vi "Auto State Machine.vi"   [LabVIEW 2013]
uses:
  typedefs/fg_typedef.ctl
  typedefs/State Machine/singleUseSubstate.ctl
  typedefs/Vision/vision enable.ctl
  typedefs/DevRef Type.ctl
  typedefs/State Machine/subStates.ctl
panel:
  # "A State Machine to Handle One or Two Ball Autonomous"
types:
  T1 = typedef "fg_typedef.ctl" = enum16{"Get", "Set"}
  T2 = typedef "subStates.ctl" = enum16{"null", "wait", "driver control", "auto", "manual override", "hold position", "rotate", "pickup", "pass", "recover pass", "load", "goto shoot", "shoot high goal", "shoot low goal", "cancel arm", "cancel shooter", "end", "test"}
  T3 = typedef "singleUseSubstate.ctl" = enum16{"null", "wait", "shift high", "shift low", "extend shooter", "retract shooter", "latch", "unlatch", "end"}
  T4 = typedef "vision enable.ctl" = enum16{"Enable", "Disable", "Stop"}
  T5 = typedef "DevRef Type.ctl" = enum16{"Shooter Solenoid", "Latch Solenoid", "Right Up Sensor", "Right Down Sensor", "Hold Sensor", "Arm Encoder"}
  T6 = typedef "WPI_EncoderDevRef.ctl" = cluster{"DevStatus":errorcluster, "EncoderIndex":T7, "CounterIndex":T8, "DistancePerCount":dbl, "Decoding Type":T9}
  T7 = typedef "FPGA_EncoderIdx.ctl" = enum8{"Enc 0", "Enc 1", "Enc 2", "Enc 3", "Invalid"}
  T8 = typedef "FPGA_CounterCtrSystemIndex.ctl" = enum8{"Ctr 0", "Ctr 1", "Ctr 2", "Ctr 3", "Ctr 4", "Ctr 5", "Ctr 6", "Ctr 7", "Invalid"}
  T9 = typedef "WPI_EncoderType.ctl" = enum16{"1x", "2x", "4x"}
  T10 = typedef "WPI_DigitalInputDevRef.ctl" = cluster{"DevStatus":errorcluster, "DIO Channel":T11, "Digital Module":T12}
  T11 = typedef "FPGA_DIOChannel.ctl" = enum8{"DIO 1", "DIO 2", "DIO 3", "DIO 4", "DIO 5", "DIO 6", "DIO 7", "DIO 8", "DIO 9", "DIO 10", "DIO 11", "DIO 12", "DIO 13", "DIO 14", "Invalid"}
  T12 = typedef "FPGA_TypedefDigitalModule.ctl" = enum16{"Digital Module 1", "Digital Module 2"}
  T13 = typedef "vision data.ctl" = cluster{"x":dbl, "y":dbl, "area":dbl, "width":dbl, "height":dbl, "Hot Goal Present?":bool, "distance":dbl}
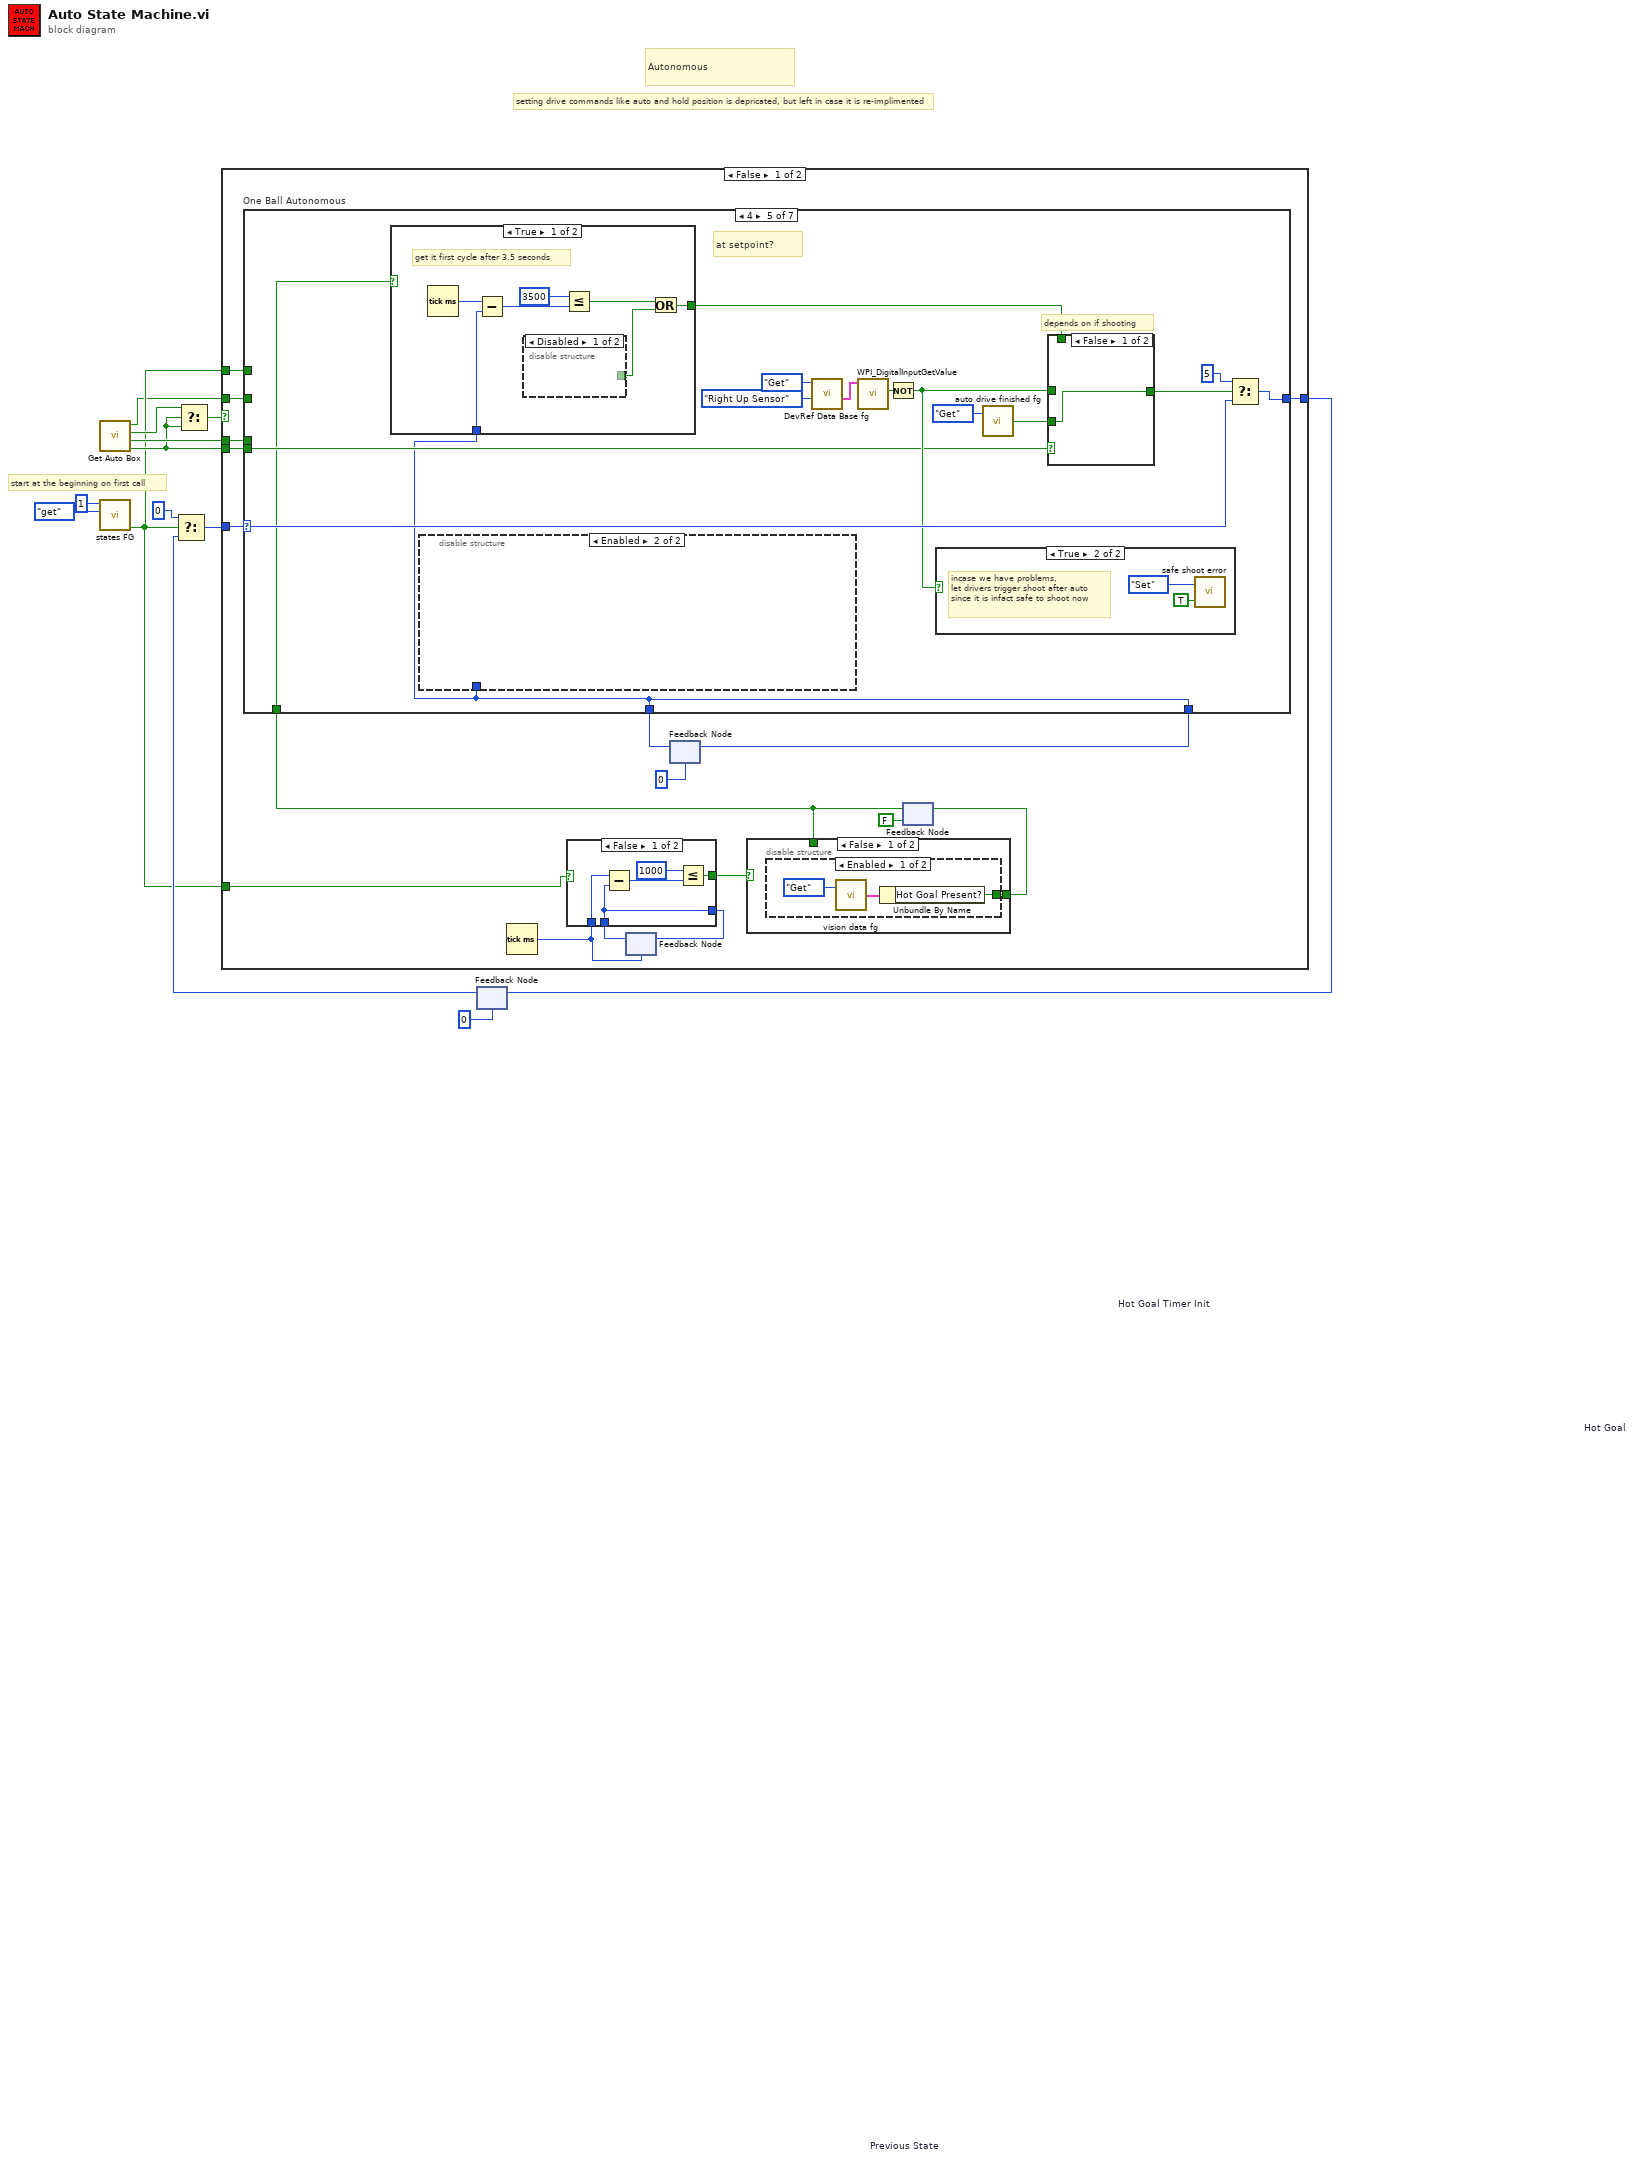
[diagram p0: block diagram]
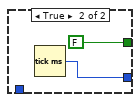
[diagram p2: hidden frame]
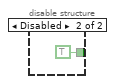
[diagram p3: hidden frame]
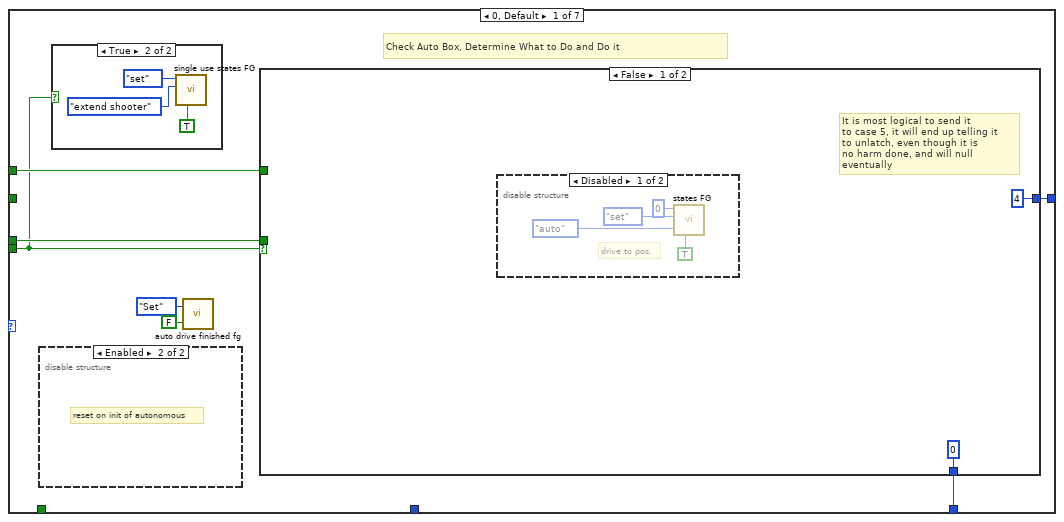
[diagram p5: hidden frame]
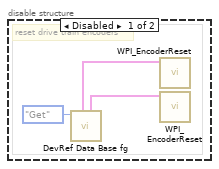
[diagram p6: hidden frame]
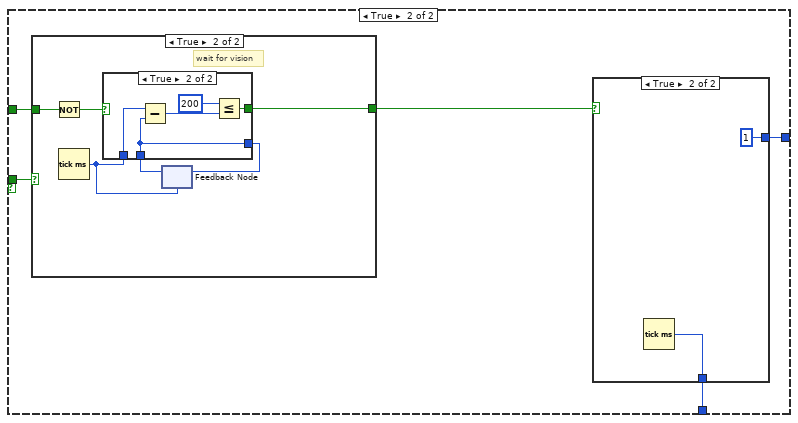
[diagram p8: hidden frame]
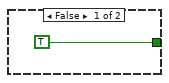
[diagram p9: hidden frame]
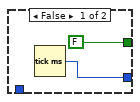
[diagram p10: hidden frame]
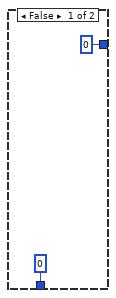
[diagram p11: hidden frame]
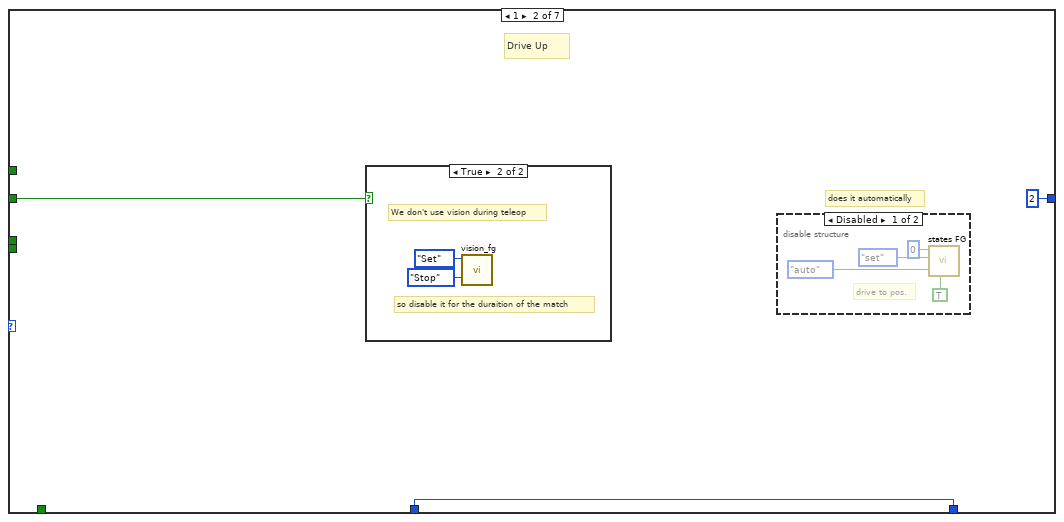
[diagram p13: hidden frame]
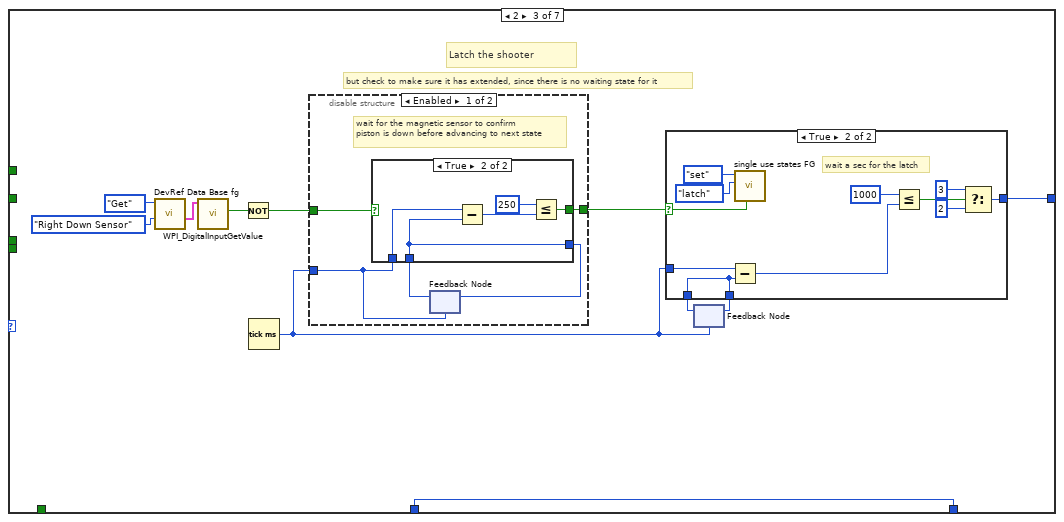
[diagram p16: hidden frame]
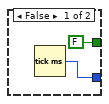
[diagram p17: hidden frame]
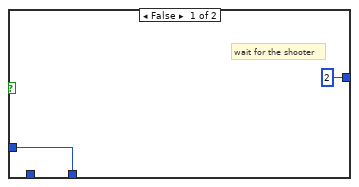
[diagram p19: hidden frame]
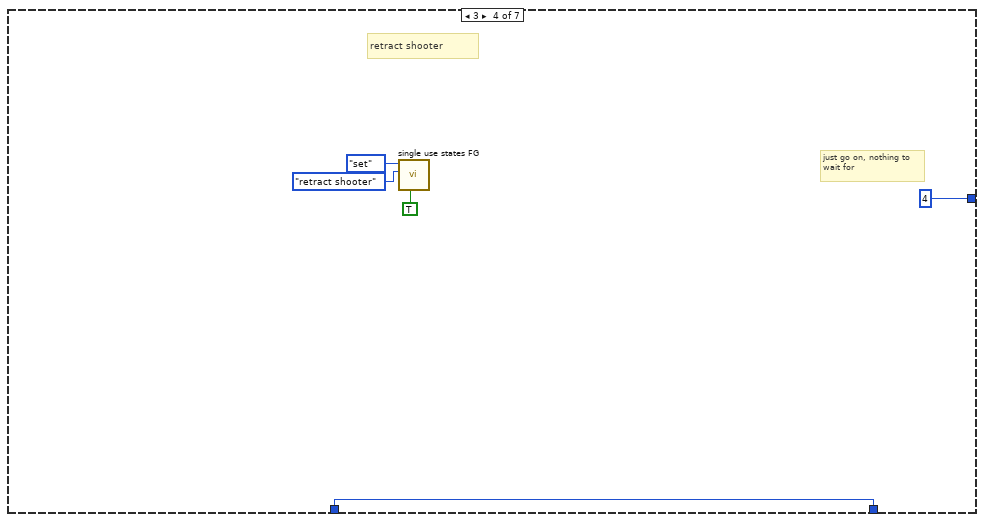
[diagram p20: hidden frame]
diagram:
  # "setting drive commands like auto and hold position is depricated, but left in case it is re-implimented"
  # "start at the beginning on first call"
  # "Autonomous"
  n1 = call "Get Auto Box.vi"() -> ("Shoot During Autonomous?"=w3:bool, "Use Hot Goal?"=w6:bool, "2 Ball Autonomous?"=w4:bool, "Disable Vison After Auto?"=w1:bool)
  n2 = call "states FG.vi"("menu (get)"=enum16{"set", "get"}."get", "Loop ID"=1) -> ("first call?"=w2:bool)  [unwired: 6 in, 3 out]
  n3 = Select(t=w4, s=w3, f=w3) -> (s? t:f=w5:bool)
  n4 = feedback #1 "Previous State"(u8 0) -> (w9:u8)
  n5 = Select(t=u8 0, s=w2, f=w9) -> (s? t:f=w11:u8)
  n6 = case shown="False" w5 {
    tunnel: w11 -> [w30 w221]
    tunnel: [w29 w214] -> w7
    tunnel: w2 -> [w27 w210]
    tunnel: w3 -> [w26 _]
    tunnel: w6 -> [w25 _]
    tunnel: w2 -> [w17 w218]
    tunnel: w1 -> [w23 _]
    frame False {
      n7 = Tick Count (ms)() -> (millisecond timer value=w15:u32)
      n8 = feedback #2(w15) -> (w20:u32)
      n9 = case shown="False" w17 {
        tunnel: [w32 w37] -> w19
        tunnel: w20 -> [w32 _]
        tunnel: [w33 FALSE] -> w18
        tunnel: w15 -> [w31 _]
        frame False {
          n10 = Subtract(x=w31, y=w32) -> (x-y=w35:u32)
          n11 = Less Or Equal?(x=u32 1000, y=w35) -> (x <= y?=w33:bool)
        }
        frame True {
          n12 = Tick Count (ms)() -> (millisecond timer value=w37:u32)
        }
      }
      n13 = feedback-in #2(w19) -> ()
      n14 = feedback #3 "Hot Goal Timer Init"(u32 0 ("millisecond timer value")) -> (w16:u32)
      n15 = feedback #4 "Hot Goal"(FALSE ("Hot Goal Present?")) -> (w14:bool)
      n16 = case "One Ball Autonomous" shown="4" w30 {
        selector: w30 -> [_ _ _ _ w151 _ w209]
        tunnel: [w50 u8 2 ("t") w101 u8 4 ("t") w149 u8 6 ("t") w209] -> w29
        tunnel: w16 -> [_ w88 w95 w132 w139 w185 w192]
        tunnel: w27 -> [w49 _ _ _ _ _ _]
        tunnel: w26 -> [w47 _ _ _ w142 _ _]
        tunnel: w25 -> [w48 _ _ _ _ _ _]
        tunnel: [w46 w88 w95 w132 w139 w185 w192] -> w24
        tunnel: w23 -> [_ w86 _ _ _ _ _]
        tunnel: w14 -> [_ _ _ _ w141 _ _]
        frame 0, Default {
          # "Check Auto Box, Determine What to Do and Do it"
          n17 = disable-structure shown="Enabled" {
            frame Disabled {
              # "reset drive train encoders"
              n18 = call "DevRef Data Base fg.vi"("Menu"=fg_typedef."Get") -> ("right drive encoder"=w51:T6, "left drive encoder"=w52:T6)  [unwired: 2 in, 7 out]
              n19 = call <vilib>:"WPI_EncoderReset.vi"("EncoderDevRef"=w52) -> ()  [unwired: 9 in, 2 out]
              n20 = call <vilib>:"WPI_EncoderReset.vi"("EncoderDevRef"=w51) -> ()  [unwired: 9 in, 2 out]
            }
            frame Enabled {
              # "reset on init of autonomous"
            }
          }
          n21 = case shown="True" w47 {
            frame False {
            }
            frame True {
              n22 = call "single use states FG.vi"("exit in"=TRUE, "substate"=singleUseSubstate."extend shooter", "menu (get)"=enum16{"set", "get"}."set") -> ()  [unwired: 5 in, 4 out]
            }
          }
          n23 = call "auto drive finished fg.vi"("Done?"=FALSE, "Menu"=fg_typedef."Set") -> ()  [unwired: 1 out]
          n24 = case shown="False" w47 {
            tunnel: [u8 4 ("f") w64] -> w50
            tunnel: w49 -> [_ w63]
            tunnel: w48 -> [_ w61]
            tunnel: [u32 0 ("millisecond timer value") w60] -> w46
            frame False {
              # "It is most logical to send it\nto case 5, it will end up telling it\nto unlatch, even though it is\nno harm done, and will null eventually"
              n25 = disable-structure shown="Disabled" {
                frame Disabled {
                  # "drive to pos."
                  n26 = call "states FG.vi"("exit in"=TRUE, "subState in"=subStates."auto", "menu (get)"=enum16{"set", "get"}."set", "Loop ID"=0) -> ()  [unwired: 4 in, 4 out]
                }
                frame Enabled {
                }
              }
            }
            frame True {
              n27 = case shown="True" w61 {
                tunnel: w63 -> [_ w71]
                tunnel: [TRUE w70] -> w62
                frame False {
                }
                frame True {
                  # "wait for vision"
                  n28 = Not(x=w71) -> (.not. x?=w66:bool)
                  n29 = Tick Count (ms)() -> (millisecond timer value=w69:u32)
                  n30 = feedback #5(w69) -> (w67:u32)
                  n31 = case shown="True" w66 {
                    tunnel: w69 -> [_ w76]
                    tunnel: [w73 w74] -> w68
                    tunnel: w67 -> [_ w74]
                    tunnel: [FALSE w75] -> w70
                    frame False {
                      n32 = Tick Count (ms)() -> (millisecond timer value=w73:u32)
                    }
                    frame True {
                      n33 = Subtract(x=w76, y=w74) -> (x-y=w78:u32)
                      n34 = Less Or Equal?(x=u32 200, y=w78) -> (x <= y?=w75:bool)
                    }
                  }
                  n35 = feedback-in #5(w68) -> ()
                }
              }
              n36 = case shown="True" w62 {
                tunnel: [u8 0 ("f") u8 1 ("f")] -> w64
                tunnel: [u32 0 ("millisecond timer value") w81] -> w60
                frame False {
                }
                frame True {
                  n37 = Tick Count (ms)() -> (millisecond timer value=w81:u32)
                }
              }
            }
          }
        }
        frame 1 {
          # "does it automatically"
          # "Drive Up"
          n38 = case shown="True" w86 {
            frame False {
            }
            frame True {
              # "so disable it for the duraition of the match"
              # "We don't use vision during teleop"
              n39 = call "vision_fg.vi"("Action"=vision_enable."Stop", "Menu"=fg_typedef."Set" ("Enum")) -> ()  [unwired: 1 in, 2 out]
            }
          }
          n40 = disable-structure shown="Disabled" {
            frame Disabled {
              # "drive to pos."
              n41 = call "states FG.vi"("exit in"=TRUE, "subState in"=subStates."auto", "menu (get)"=enum16{"set", "get"}."set", "Loop ID"=0) -> ()  [unwired: 4 in, 4 out]
            }
            frame Enabled {
            }
          }
        }
        frame 2 {
          # "but check to make sure it has extended, since there is no waiting state for it"
          # "Latch the shooter"
          n42 = call "DevRef Data Base fg.vi"("DevRef to Get"=DevRef_Type."Right Down Sensor", "Menu"=fg_typedef."Get") -> ("Selected Sensor"=w105:T10)  [unwired: 1 in, 8 out]
          n43 = call <vilib>:"WPI_DigitalInputGetValue.vi"("DigitalInputDevRef"=w105) -> ("Value"=w104:bool)  [unwired: 8 in, 2 out]
          n44 = Not(x=w104) -> (.not. x?=w98:bool)
          n45 = Tick Count (ms)() -> (millisecond timer value=w97:u32)
          n46 = disable-structure shown="Enabled" {
            disable-tunnel: w98 -> [w110 w118]
            disable-tunnel: [w107 w118] -> w96
            disable-tunnel: w97 -> [w106 _]
            frame Enabled {
              # "wait for the magnetic sensor to confirm \npiston is down before advancing to next state"
              n47 = feedback #6(w106) -> (w108:u32)
              n48 = case shown="True" w110 {
                tunnel: w106 -> [_ w115]
                tunnel: [w112 w113] -> w109
                tunnel: w108 -> [_ w113]
                tunnel: [FALSE w114] -> w107
                frame False {
                  n49 = Tick Count (ms)() -> (millisecond timer value=w112:u32)
                }
                frame True {
                  n50 = Subtract(x=w115, y=w113) -> (x-y=w117:u32)
                  n51 = Less Or Equal?(x=u32 250, y=w117) -> (x <= y?=w114:bool)
                }
              }
              n52 = feedback-in #6(w109) -> ()
            }
            frame Disabled {
            }
          }
          n53 = feedback #7(w97) -> (w102:u32)
          n54 = case shown="True" w96 {
            selector: w96 -> [_ w127]
            tunnel: [w119 w129] -> w103
            tunnel: w102 -> [_ w129]
            tunnel: w97 -> [w119 w128]
            tunnel: [u8 2 ("f") w122] -> w101
            frame False {
              # "wait for the shooter"
            }
            frame True {
              # "wait a sec for the latch"
              n55 = Subtract(x=w128, y=w129) -> (x-y=w124:u32)
              n56 = call "single use states FG.vi"("exit in"=w127, "substate"=singleUseSubstate."latch", "menu (get)"=enum16{"set", "get"}."set") -> ()  [unwired: 5 in, 4 out]
              n57 = Less Or Equal?(x=u32 1000, y=w124) -> (x <= y?=w121:bool)
              n58 = Select(t=u8 3, s=w121, f=u8 2) -> (s? t:f=w122:u8)
            }
          }
          n59 = feedback-in #7(w103) -> ()
        }
        frame 3 {
          # "just go on, nothing to\nwait for"
          # "retract shooter"
          n60 = call "single use states FG.vi"("exit in"=TRUE, "substate"=singleUseSubstate."retract shooter", "menu (get)"=enum16{"set", "get"}."set") -> ()  [unwired: 5 in, 4 out]
        }
        frame 4 {
          # "depends on if shooting"
          # "at setpoint?"
          n61 = case shown="True" w141 {
            tunnel: w139 -> [w168 w174]
            tunnel: [w167 w173] -> w140
            frame True {
              # "get it first cycle after 3.5 seconds"
              n62 = Tick Count (ms)() -> (millisecond timer value=w169:u32)
              n63 = Subtract(x=w169, y=w168) -> (x-y=w171:u32)
              n64 = disable-structure shown="Disabled" {
                disable-tunnel: [_ FALSE ("Done")] -> w165
                frame Disabled {
                }
                frame Enabled {
                }
              }
              n65 = Less Or Equal?(x=u32 3500, y=w171) -> (x <= y?=w166:bool)
              n66 = Or(x=w166, y=w165) -> (x .or. y?=w167:bool)
            }
            frame False {
              # "wait 5.25 seconds for hot goal to switch"
              n67 = Tick Count (ms)() -> (millisecond timer value=w175:u32)
              n68 = Subtract(x=w175, y=w174) -> (x-y=w177:u32)
              n69 = Less Or Equal?(x=u32 5250, y=w177) -> (x <= y?=w173:bool)
            }
          }
          n70 = disable-structure shown="Enabled" {
            disable-tunnel: w139 -> [w154 _]
            frame Disabled {
              n71 = Tick Count (ms)() -> (millisecond timer value=w157:u32)
              n72 = Subtract(x=w157, y=w154) -> (x-y=w155:u32)
              n73 = Less Or Equal?(x=u32 4100, y=w155) -> (x <= y?=w153:bool)
              n74 = disable-structure shown="Enabled" {
                disable-tunnel: w153 -> [w159 _]
                disable-tunnel: fg_typedef."Set" ("Menu") -> [w158 _]
                frame Enabled {
                  n75 = case shown="True" w159 {
                    selector: w159 -> [_ w161]
                    tunnel: w158 -> [_ w160]
                    frame False {
                    }
                    frame True {
                      n76 = call "auto drive finished fg.vi"("Done?"=w161, "Menu"=w160) -> ()  [unwired: 1 out]
                      n77 = call "states FG.vi"("exit in"=w161, "subState in"=subStates."null" ("y"), "menu (get)"=enum16{"set", "get"}."set", "Loop ID"=0) -> ()  [unwired: 4 in, 4 out]
                    }
                  }
                }
                frame Disabled {
                }
              }
            }
            frame Enabled {
            }
          }
          n78 = call "DevRef Data Base fg.vi"("DevRef to Get"=DevRef_Type."Right Up Sensor", "Menu"=fg_typedef."Get") -> ("Selected Sensor"=w148:T10)  [unwired: 1 in, 8 out]
          n79 = call <vilib>:"WPI_DigitalInputGetValue.vi"("DigitalInputDevRef"=w148) -> ("Value"=w147:bool)  [unwired: 8 in, 2 out]
          n80 = Not(x=w147) -> (.not. x?=w144:bool)
          n81 = case shown="True" w144 {
            frame False {
            }
            frame True {
              # "incase we have problems,\nlet drivers trigger shoot after auto\nsince it is infact safe to shoot now"
              n82 = call "safe shoot error.vi"("Can Shoot Safely?"=TRUE, "Menu"=fg_typedef."Set") -> ()  [unwired: 1 out]
            }
          }
          n83 = call "auto drive finished fg.vi"("Menu"=fg_typedef."Get") -> ("Done"=w137:bool)  [unwired: 1 in]
          n84 = case shown="False" w142 {
            tunnel: w140 -> [_ w182]
            tunnel: w144 -> [_ w181]
            tunnel: w137 -> [w178 w180]
            tunnel: [w178 w179] -> w143
            frame False {
            }
            frame True {
              n85 = Compound Arithmetic op=AND(w182, w181, w180) -> (w179:bool)
            }
          }
          n86 = Select(t=u8 5, s=w143, f=w151) -> (s? t:f=w149:u8)
        }
        frame 5 {
          w188 = FALSE ("Can Shoot Safely?")
          w187 = fg_typedef."Set" ("Menu")
          # "unlatch shooter"
          # "SHOOT!!!"
          n87 = call "safe shoot error.vi"("Can Shoot Safely?"=w188, "Menu"=w187) -> ()  [unwired: 1 out]
          n88 = call "auto drive finished fg.vi"("Done?"=w188, "Menu"=w187) -> ()  [unwired: 1 out]
          n89 = call "single use states FG.vi"("exit in"=TRUE, "substate"=singleUseSubstate."unlatch", "menu (get)"=enum16{"set", "get"}."set") -> ()  [unwired: 5 in, 4 out]
        }
        frame 6 {
          # "null things"
          # "null all the things"
          n90 = call "states FG.vi"("exit in"=TRUE, "subState in"=subStates."null", "menu (get)"=enum16{"set", "get"}."set", "Loop ID"=0) -> ()  [unwired: 4 in, 4 out]
          n91 = call "states FG.vi"("exit in"=TRUE, "subState in"=subStates."null", "menu (get)"=enum16{"set", "get"}."set", "Loop ID"=1) -> ()  [unwired: 4 in, 4 out]
          n92 = call "states FG.vi"("exit in"=TRUE, "subState in"=subStates."null", "menu (get)"=enum16{"set", "get"}."set", "Loop ID"=2) -> ()  [unwired: 4 in, 4 out]
          n93 = call "states FG.vi"("exit in"=TRUE, "subState in"=subStates."null", "menu (get)"=enum16{"set", "get"}."set", "Loop ID"=3) -> ()  [unwired: 4 in, 4 out]
        }
      }
      n94 = feedback-in #3(w24) -> ()
      n95 = case shown="False" w18 {
        tunnel: [w38 w43] -> w21
        tunnel: w14 -> [_ w43]
        frame False {
          n96 = disable-structure shown="Enabled" {
            disable-tunnel: [w39 TRUE ("Hot Goal Present?")] -> w38
            frame Enabled {
              n97 = call "vision data fg.vi"("Menu"=fg_typedef."Get") -> ("Output"=w41:T13)  [unwired: 1 in]
              n98 = Unbundle By Name(w41) -> ("Hot Goal Present?"=w39:bool)
            }
            frame Disabled {
            }
          }
        }
        frame True {
        }
      }
      n99 = feedback-in #4(w21) -> ()
    }
    frame True {
      n100 = feedback #8 "Wait Timer Init"(u32 0 ("millisecond timer value")) -> (w211:u32)
      n101 = case "Two Ball Autonomous" shown="0, Default" w221 {
        selector: w221 -> [_ w298 _ w317 _ w351 _ _ w372 w410 _ w428]
        tunnel: [u8 1 ("t") w300 u8 3 ("t") w314 u8 5 ("t") w353 u8 7 ("t") u8 8 ("t") w373 w409 u8 11 ("t") w428] -> w214
        tunnel: [_ _ w308 w315 _ _ _ _ _ _ _ _] -> w212
        tunnel: w211 -> [_ _ _ w316 _ _ _ _ _ _ _ _]
        tunnel: w210 -> [w279 _ _ _ _ _ _ _ _ _ _ _]
        frame 0, Default {
          # "full reverse is belts in"
          # "belts on"
          # "up setpoint"
          # "put arm out"
          # "Arm Up, Belts In"
          # "reset drive train encoders"
          n102 = case shown="True" w279 {
            frame False {
            }
            frame True {
              # "so disable it for the duraition of the match"
              # "We don't use vision during teleop"
              n103 = call "vision_fg.vi"("Action"=vision_enable."Stop", "Menu"=fg_typedef."Set" ("Enum")) -> ()  [unwired: 1 in, 2 out]
            }
          }
          n104 = call "auto drive finished fg.vi"("Done?"=FALSE, "Menu"=fg_typedef."Set") -> ()  [unwired: 1 out]
          n105 = call "Arm Setpoint FG.vi"("Setpoint In"=55.0, "Menu"=fg_typedef."Set") -> ()  [unwired: 1 out]
          n106 = call "states FG.vi"("exit in"=TRUE, "subState in"=subStates."auto", "menu (get)"=enum16{"set", "get"}."set", "Loop ID"=3) -> ()  [unwired: 4 in, 4 out]
          n107 = call "Belt Speed FG.vi"("Speed In"=-1.0 ("Setpoint In"), "Menu"=fg_typedef."Set") -> ()  [unwired: 1 out]
          n108 = call "states FG.vi"("exit in"=TRUE, "subState in"=subStates."auto", "menu (get)"=enum16{"set", "get"}."set", "Loop ID"=2) -> ()  [unwired: 4 in, 4 out]
          n109 = call "DevRef Data Base fg.vi"("Menu"=fg_typedef."Get") -> ("right drive encoder"=w293:T6, "left drive encoder"=w294:T6)  [unwired: 2 in, 7 out]
          n110 = call <vilib>:"WPI_EncoderReset.vi"("EncoderDevRef"=w294) -> ()  [unwired: 9 in, 2 out]
          n111 = call <vilib>:"WPI_EncoderReset.vi"("EncoderDevRef"=w293) -> ()  [unwired: 9 in, 2 out]
        }
        frame 1 {
          # "Wait for Arm"
          n112 = call "DevRef Data Base fg.vi"("DevRef to Get"=DevRef_Type."Arm Encoder", "Menu"=fg_typedef."Get") -> ("Selected Encoder"=w307:T6)  [unwired: 1 in, 8 out]
          n113 = call <vilib>:"WPI_EncoderGet.vi"("EncoderDevRef"=w307) -> ("Distance"=w306:dbl)  [unwired: 5 in, 5 out]
          n114 = In Range and Coerce(upper limit=55.0, x=w306, lower limit=45.0) -> (In Range?=w299:bool)  [unwired: 1 out]
          n115 = Select(t=u8 2, s=w299, f=w298) -> (s? t:f=w300:u8)
        }
        frame 2 {
          # "drive to reverse position"
          n116 = Tick Count (ms)() -> (millisecond timer value=w308:u32)
          n117 = call "states FG.vi"("exit in"=TRUE, "subState in"=subStates."auto", "menu (get)"=enum16{"set", "get"}."set", "Loop ID"=0) -> ()  [unwired: 4 in, 4 out]
        }
        frame 3 {
          # "Wait for Ball"
          n118 = disable-structure shown="Enabled" {
            disable-tunnel: w317 -> [w319 w328]
            disable-tunnel: w316 -> [_ w330]
            disable-tunnel: [_ w330] -> w315
            disable-tunnel: [w318 w326] -> w314
            frame Disabled {
              n119 = call "DevRef Data Base fg.vi"("DevRef to Get"=DevRef_Type."Hold Sensor", "Menu"=fg_typedef."Get") -> ("Selected Sensor"=w323:T10)  [unwired: 1 in, 8 out]
              n120 = call <vilib>:"WPI_DigitalInputGetValue.vi"("DigitalInputDevRef"=w323) -> ("Value"=w325:bool)  [unwired: 8 in, 2 out]
              n121 = Not(x=w325) -> (.not. x?=w324:bool)
              n122 = Select(t=u8 4, s=w324, f=w319) -> (s? t:f=w318:u8)
            }
            frame Enabled {
              n123 = Tick Count (ms)() -> (millisecond timer value=w333:u32)
              n124 = Subtract(x=w333, y=w330) -> (x-y=w332:u32)
              n125 = Less Or Equal?(x=u32 1000, y=w332) -> (x <= y?=w329:bool)
              n126 = Select(t=u8 4, s=w329, f=w328) -> (s? t:f=w326:u8)
            }
          }
        }
        frame 4 {
          # "drive to forward position"
          # "arm rests on ball"
          # "reset fg"
          # "reset fg"
          # "Belts Off, Arm Hold Ball"
          n127 = call "states FG.vi"("exit in"=TRUE, "subState in"=subStates."auto", "menu (get)"=enum16{"set", "get"}."set", "Loop ID"=0) -> ()  [unwired: 4 in, 4 out]
          n128 = call "Belt Speed FG.vi"("Speed In"=0.0 ("Setpoint In"), "Menu"=fg_typedef."Set") -> ()  [unwired: 1 out]
          n129 = call "states FG.vi"("exit in"=TRUE, "subState in"=subStates."null", "menu (get)"=enum16{"set", "get"}."set", "Loop ID"=3) -> ()  [unwired: 4 in, 4 out]
          n130 = call "states FG.vi"("exit in"=TRUE, "subState in"=subStates."null", "menu (get)"=enum16{"set", "get"}."set", "Loop ID"=2) -> ()  [unwired: 4 in, 4 out]
          n131 = call "Arm Setpoint FG.vi"("Setpoint In"=0.0, "Menu"=fg_typedef."Set") -> ()  [unwired: 1 out]
        }
        frame 5 {
          w357 = fg_typedef."Get" ("Menu")
          # "Ready to Shoot 1st Ball?"
          n132 = call "safe shoot error.vi"("Menu"=w357) -> ("Can Shoot Safely?"=w356:bool)  [unwired: 1 in]
          n133 = call "auto drive finished fg.vi"("Menu"=w357) -> ("Done"=w355:bool)  [unwired: 1 in]
          n134 = And(x=w356, y=w355) -> (x .and. y?=w352:bool)
          n135 = Select(t=u8 6, s=w352, f=w351) -> (s? t:f=w353:u8)
        }
        frame 6 {
          w360 = FALSE ("Can Shoot Safely?")
          w359 = fg_typedef."Set" ("Menu")
          # "unlatch shooter"
          # "stop driving"
          n136 = call "states FG.vi"("exit in"=TRUE, "subState in"=subStates."hold position", "menu (get)"=enum16{"set", "get"}."set", "Loop ID"=0) -> ()  [unwired: 4 in, 4 out]
          n137 = call "safe shoot error.vi"("Can Shoot Safely?"=w360, "Menu"=w359) -> ()  [unwired: 1 out]
          n138 = call "auto drive finished fg.vi"("Done?"=w360, "Menu"=w359) -> ()  [unwired: 1 out]
          n139 = call "single use states FG.vi"("exit in"=TRUE, "substate"=singleUseSubstate."unlatch", "menu (get)"=enum16{"set", "get"}."set") -> ()  [unwired: 5 in, 4 out]
        }
        frame 7 {
          # "Cock again"
          # "extend shooter"
          n140 = call "single use states FG.vi"("exit in"=TRUE, "substate"=singleUseSubstate."extend shooter", "menu (get)"=enum16{"set", "get"}."set") -> ()  [unwired: 5 in, 4 out]
        }
        frame 8 {
          # "Wait to Latch Shooter, Then Latch"
          n141 = call "DevRef Data Base fg.vi"("DevRef to Get"=DevRef_Type."Right Down Sensor", "Menu"=fg_typedef."Get") -> ("Selected Sensor"=w375:T10)  [unwired: 1 in, 8 out]
          n142 = call <vilib>:"WPI_DigitalInputGetValue.vi"("DigitalInputDevRef"=w375) -> ("Value"=w374:bool)  [unwired: 8 in, 2 out]
          n143 = Tick Count (ms)() -> (millisecond timer value=w382:u32)
          n144 = Not(x=w374) -> (.not. x?=w378:bool)
          n145 = disable-structure shown="Enabled" {
            disable-tunnel: w378 -> [w400 w408]
            disable-tunnel: [w397 w408] -> w381
            disable-tunnel: w382 -> [w396 _]
            frame Enabled {
              # "wait for the magnetic sensor to confirm \npiston is down before advancing to next state"
              n146 = feedback #9(w396) -> (w398:u32)
              n147 = case shown="True" w400 {
                tunnel: w396 -> [_ w405]
                tunnel: [w402 w403] -> w399
                tunnel: w398 -> [_ w403]
                tunnel: [FALSE w404] -> w397
                frame False {
                  n148 = Tick Count (ms)() -> (millisecond timer value=w402:u32)
                }
                frame True {
                  n149 = Subtract(x=w405, y=w403) -> (x-y=w407:u32)
                  n150 = Less Or Equal?(x=u32 250, y=w407) -> (x <= y?=w404:bool)
                }
              }
              n151 = feedback-in #9(w399) -> ()
            }
            frame Disabled {
            }
          }
          n152 = feedback #10(w382) -> (w380:u32)
          n153 = case shown="True" w381 {
            selector: w381 -> [_ w391]
            tunnel: [w384 w393] -> w379
            tunnel: w380 -> [_ w393]
            tunnel: w382 -> [w384 w392]
            tunnel: [w383 w387] -> w373
            tunnel: w372 -> [w383 w385]
            frame False {
              # "wait for the shooter"
            }
            frame True {
              # "wait a sec for the latch"
              n154 = Subtract(x=w392, y=w393) -> (x-y=w388:u32)
              n155 = call "single use states FG.vi"("exit in"=w391, "substate"=singleUseSubstate."latch", "menu (get)"=enum16{"set", "get"}."set") -> ()  [unwired: 5 in, 4 out]
              n156 = Less Or Equal?(x=u32 1000, y=w388) -> (x <= y?=w386:bool)
              n157 = Select(t=u8 9, s=w386, f=w385) -> (s? t:f=w387:u8)
            }
          }
          n158 = feedback-in #10(w379) -> ()
        }
        frame 9 {
          # "Retract Shooter"
          # "retract shooter"
          n159 = call "single use states FG.vi"("exit in"=TRUE, "substate"=singleUseSubstate."retract shooter", "menu (get)"=enum16{"set", "get"}."set") -> ()  [unwired: 5 in, 4 out]
          n160 = call "DevRef Data Base fg.vi"("DevRef to Get"=DevRef_Type."Right Up Sensor", "Menu"=fg_typedef."Get") -> ("Selected Sensor"=w411:T10)  [unwired: 1 in, 8 out]
          n161 = call <vilib>:"WPI_DigitalInputGetValue.vi"("DigitalInputDevRef"=w411) -> ("Value"=w412:bool)  [unwired: 8 in, 2 out]
          n162 = Not(x=w412) -> (.not. x?=w416:bool)
          n163 = case shown="True" w416 {
            frame False {
            }
            frame True {
              # "incase we have problems,\nlet drivers trigger shoot after auto\nsince it is infact safe to shoot now"
              n164 = call "safe shoot error.vi"("Can Shoot Safely?"=TRUE, "Menu"=fg_typedef."Set") -> ()  [unwired: 1 out]
            }
          }
          n165 = Select(t=u8 10, s=w416, f=w410) -> (s? t:f=w409:u8)
        }
        frame 10 {
          w424 = FALSE ("Can Shoot Safely?")
          w423 = fg_typedef."Set" ("Menu")
          # "unlatch shooter"
          # "Shoot Second Ball"
          n166 = call "safe shoot error.vi"("Can Shoot Safely?"=w424, "Menu"=w423) -> ()  [unwired: 1 out]
          n167 = call "auto drive finished fg.vi"("Done?"=w424, "Menu"=w423) -> ()  [unwired: 1 out]
          n168 = call "single use states FG.vi"("exit in"=TRUE, "substate"=singleUseSubstate."unlatch", "menu (get)"=enum16{"set", "get"}."set") -> ()  [unwired: 5 in, 4 out]
        }
        frame 11 {
          # "Null Everything"
          # "null things"
          n169 = call "states FG.vi"("exit in"=TRUE, "subState in"=subStates."null", "menu (get)"=enum16{"set", "get"}."set", "Loop ID"=0) -> ()  [unwired: 4 in, 4 out]
          n170 = call "states FG.vi"("exit in"=TRUE, "subState in"=subStates."null", "menu (get)"=enum16{"set", "get"}."set", "Loop ID"=1) -> ()  [unwired: 4 in, 4 out]
          n171 = call "states FG.vi"("exit in"=TRUE, "subState in"=subStates."null", "menu (get)"=enum16{"set", "get"}."set", "Loop ID"=2) -> ()  [unwired: 4 in, 4 out]
          n172 = call "states FG.vi"("exit in"=TRUE, "subState in"=subStates."null", "menu (get)"=enum16{"set", "get"}."set", "Loop ID"=3) -> ()  [unwired: 4 in, 4 out]
        }
      }
      n173 = feedback-in #8(w212) -> ()
      n174 = feedback #11 "Previous State"(u8 0) -> (w216:u8)
      n175 = Select(t=u8 0, s=w218, f=w216) -> (s? t:f=w219:u8)
      n176 = case "Parallel Initial Pneumatics" shown="0, Default" w219 {
        selector: w219 -> [_ w226 w273 w276]
        tunnel: [u8 1 ("t") w229 w264 w276] -> w215
        frame 0, Default {
          # "Cock Shooter for Pre-Loaded Ball"
          # "extend shooter"
          n177 = call "single use states FG.vi"("exit in"=TRUE, "substate"=singleUseSubstate."extend shooter", "menu (get)"=enum16{"set", "get"}."set") -> ()  [unwired: 5 in, 4 out]
        }
        frame 1 {
          # "Wait to Latch Shooter, Then Latch"
          n178 = call "DevRef Data Base fg.vi"("DevRef to Get"=DevRef_Type."Right Down Sensor", "Menu"=fg_typedef."Get") -> ("Selected Sensor"=w235:T10)  [unwired: 1 in, 8 out]
          n179 = call <vilib>:"WPI_DigitalInputGetValue.vi"("DigitalInputDevRef"=w235) -> ("Value"=w236:bool)  [unwired: 8 in, 2 out]
          n180 = Tick Count (ms)() -> (millisecond timer value=w227:u32)
          n181 = Not(x=w236) -> (.not. x?=w232:bool)
          n182 = disable-structure shown="Enabled" {
            disable-tunnel: w232 -> [w254 w262]
            disable-tunnel: [w251 w262] -> w228
            disable-tunnel: w227 -> [w250 _]
            frame Enabled {
              # "wait for the magnetic sensor to confirm \npiston is down before advancing to next state"
              n183 = feedback #12(w250) -> (w252:u32)
              n184 = case shown="True" w254 {
                tunnel: w250 -> [_ w259]
                tunnel: [w256 w257] -> w253
                tunnel: w252 -> [_ w257]
                tunnel: [FALSE w258] -> w251
                frame False {
                  n185 = Tick Count (ms)() -> (millisecond timer value=w256:u32)
                }
                frame True {
                  n186 = Subtract(x=w259, y=w257) -> (x-y=w261:u32)
                  n187 = Less Or Equal?(x=u32 250, y=w261) -> (x <= y?=w258:bool)
                }
              }
              n188 = feedback-in #12(w253) -> ()
            }
            frame Disabled {
            }
          }
          n189 = feedback #13(w227) -> (w230:u32)
          n190 = case shown="True" w228 {
            selector: w228 -> [_ w245]
            tunnel: [w238 w247] -> w231
            tunnel: w230 -> [_ w247]
            tunnel: w227 -> [w238 w246]
            tunnel: [w237 w241] -> w229
            tunnel: w226 -> [w237 w239]
            frame False {
              # "wait for the shooter"
            }
            frame True {
              # "wait a sec for the latch"
              n191 = Subtract(x=w246, y=w247) -> (x-y=w242:u32)
              n192 = call "single use states FG.vi"("exit in"=w245, "substate"=singleUseSubstate."latch", "menu (get)"=enum16{"set", "get"}."set") -> ()  [unwired: 5 in, 4 out]
              n193 = Less Or Equal?(x=u32 1000, y=w242) -> (x <= y?=w240:bool)
              n194 = Select(t=u8 2, s=w240, f=w239) -> (s? t:f=w241:u8)
            }
          }
          n195 = feedback-in #13(w231) -> ()
        }
        frame 2 {
          # "retract shooter"
          # "Retract Shooter"
          n196 = call "single use states FG.vi"("exit in"=TRUE, "substate"=singleUseSubstate."retract shooter", "menu (get)"=enum16{"set", "get"}."set") -> ()  [unwired: 5 in, 4 out]
          n197 = call "DevRef Data Base fg.vi"("DevRef to Get"=DevRef_Type."Right Up Sensor", "Menu"=fg_typedef."Get") -> ("Selected Sensor"=w269:T10)  [unwired: 1 in, 8 out]
          n198 = call <vilib>:"WPI_DigitalInputGetValue.vi"("DigitalInputDevRef"=w269) -> ("Value"=w268:bool)  [unwired: 8 in, 2 out]
          n199 = Not(x=w268) -> (.not. x?=w263:bool)
          n200 = case shown="True" w263 {
            frame False {
            }
            frame True {
              # "incase we have problems,\nlet drivers trigger shoot after auto\nsince it is infact safe to shoot now"
              n201 = call "safe shoot error.vi"("Can Shoot Safely?"=TRUE, "Menu"=fg_typedef."Set") -> ()  [unwired: 1 out]
            }
          }
          n202 = Select(t=u8 3, s=w263, f=w273) -> (s? t:f=w264:u8)
        }
        frame 3 {
        }
      }
      n203 = feedback-in #11(w215) -> ()
    }
  }
  n204 = feedback-in #1(w7) -> ()
